vi "Update Generation On The Fly Digital Audio Task.vi"(7 "output level units":T1, 8 "error in (no error)":errorcluster, 10 "sine wave properties":T2, 11 "data task":T3) -> (0 "error out":errorcluster, 3 "data task":T3)   [LabVIEW 2021, in "DigitalAudioGenerationProcess.lvlib"]
uses:
  DigitalAudioGenerationProcess.lvlib
  <vilib>/PDM Acquisition Toolkit/host/Classes/Tasks/PCM Output/Controls/PCM Output Task DVR.ctl
  <vilib>/PDM Acquisition Toolkit/host/Classes/Tasks/PCM Output/PCM Output Task.lvclass
  C:/Program Files/National Instruments/LabVIEW 2021/vi.lib/PDM Acquisition Toolkit/host/Classes/Tasks/Parent/DecoderTask.lvclass
  controls/sine wave properties.ctl
  <vilib>/PDM Acquisition Toolkit/host/Classes/Channels/PCM Output/PCM Output Channel.lvclass
  C:/Program Files/National Instruments/LabVIEW 2021/vi.lib/PDM Acquisition Toolkit/host/Classes/Channels/DecoderChannel.lvclass
  <vilib>/PDM Acquisition Toolkit/host/Classes/Channels/PCM Output/controls/PCM Output Channel - Signal Properties.ctl
  <vilib>/PDM Acquisition Toolkit/host/Classes/Channels/DecoderChannel.lvclass
  C:/Program Files/National Instruments/LabVIEW 2021/vi.lib/PDM Acquisition Toolkit/host/Classes/Channels/PCM Output/PCM Output Channel.lvclass
  controls/AudioGenTypeDefs.lvlib
  shared/controls/digital output level units.ctl
  shared/controls/audio controls.lvlib
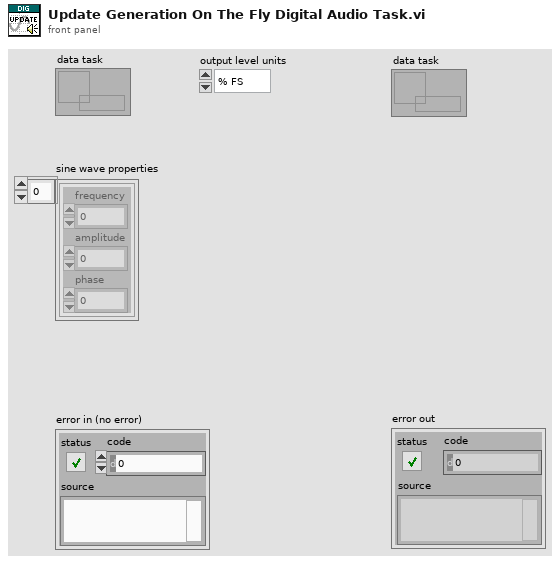
[diagram p1: front panel]
types:
  T1 = typedef "audio controls.lvlib/digital output level units.ctl" = enum32{"% FS", "dBFS", "V"}
  T2 = typedef "AudioGenTypeDefs.lvlib/sine wave properties.ctl" = cluster{"frequency":dbl, "amplitude":dbl, "phase":dbl}[]
  T3 = typedef "PDM Acquisition Class Library.lvlib/PCM Output Task.lvclass/PCM Output Task DVR.ctl" = refnum<data-value>
  T4 = typedef "PDM Acquisition Class Library.lvlib/PCM Output Channel.lvclass/PCM Output Channel - Signal Properties.ctl" = cluster{"cyclic period":dbl, "cyclic phase offset":dbl, "gain":dbl}
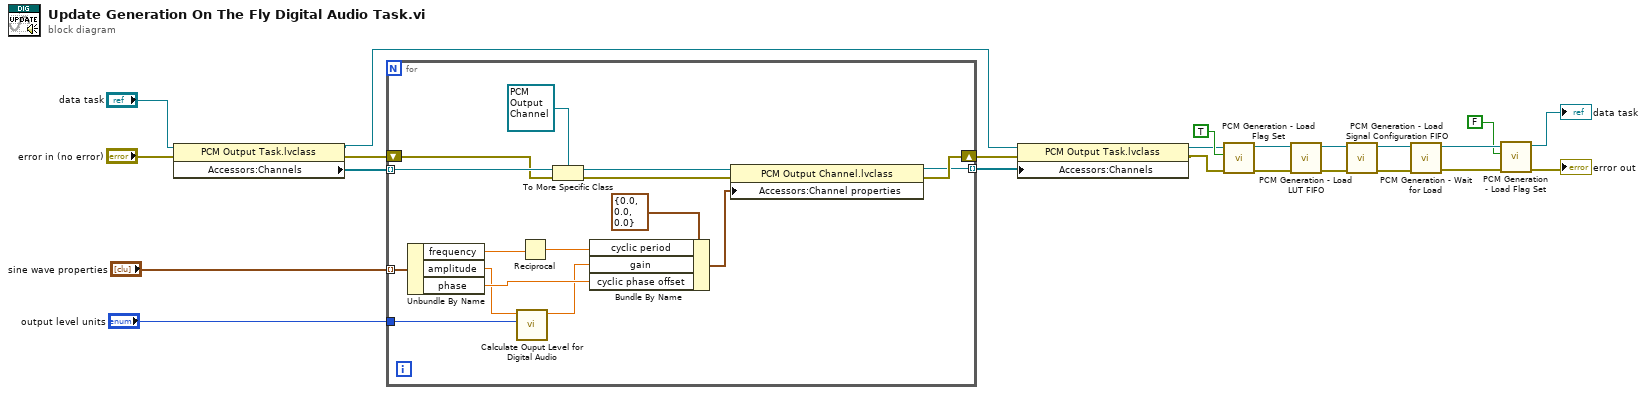
[diagram p0: block diagram]
diagram:
  n1 = property class="PCM Output Task.lvclass"(reference="data task", error in="error in (no error)") -> (reference out=w10:T3, error out=w22:errorcluster, "Accessors:Channels"=w23:refnum<class "DecoderChannel.lvclass">[])
  n2 = for {
    tunnel: w23 -> [w38] mode=indexing
    shift-right: [w34] -> w12
    shift-left: w22 -> [w36]
    tunnel: [w33] -> w11 mode=indexing
    tunnel: "sine wave properties" -> [w29] mode=indexing
    tunnel: "output level units" -> [w24]
    n3 = Unbundle By Name(w29) -> ("frequency"=w28:dbl, "amplitude"=w26:dbl, "phase"=w27:dbl)
    n4 = call "Calculate Ouput Level for Digital Audio.vi"("digital output level units"=w24, "output level"=w26) -> ("gain"=w25:dbl)  [unwired: 8 in, 1 out]
    n5 = Reciprocal(x=w28) -> (1/x=w32:dbl)
    n6 = To More Specific Class(target class=refnum<class "PCM Output Channel.lvclass"> refnum ("PDM Acquisition Class Library.lvlib:PCM Output Channel.lvclass"), reference=w38, error in=w36) -> (specific class reference=w35:refnum<class "PCM Output Channel.lvclass">, error out=w39:errorcluster)
    n7 = Bundle By Name(cluster=T4 {"cyclic period"=0.0, "cyclic phase offset"=0.0, "gain"=0.0} ("Channel properties"), "cyclic period"=w32, "gain"=w25, "cyclic phase offset"=w27) -> (w30:T4)
    n8 = property class="PCM Output Channel.lvclass"(reference=w35, error in=w39, "Accessors:Channel properties"=w30) -> (reference out=w33:refnum<class "PCM Output Channel.lvclass">, error out=w34:errorcluster)
  }
  n9 = property class="PCM Output Task.lvclass"(reference=w10, error in=w12, "Accessors:Channels"=w11) -> (reference out=w9:T3, error out=w8:errorcluster)
  n10 = call <vilib>:"PCM Generation - Load Flag Set.vi"("error in"=w8, "Load"=TRUE, "PCM Output Task In"=w9) -> ("error out"=w16:errorcluster, "PCM Output Task Out"=w15:T3)  [unwired: 7 in]
  n11 = call <vilib>:"PCM Generation - Load LUT FIFO.vi"("error in"=w16, "PCM Output Task In"=w15) -> ("error out"=w13:errorcluster, "PCM Output Task Out"=w14:T3)  [unwired: 8 in]
  n12 = call <vilib>:"PCM Generation - Load Signal Configuration FIFO.vi"("error in"=w13, "PCM Output Task In"=w14) -> ("error out"=w7:errorcluster, "PCM Output Task Out"=w17:T3)  [unwired: 8 in]
  n13 = call <vilib>:"PCM Generation - Wait for Load.vi"("error in"=w7, "PCM Output Task In"=w17) -> ("error out"=w19:errorcluster, "PCM Output Task Out"=w20:T3)  [unwired: 7 in, 1 out]
  n14 = call <vilib>:"PCM Generation - Load Flag Set.vi"("error in"=w19, "Load"=FALSE, "PCM Output Task In"=w20) -> ("error out"=→"error out":errorcluster, "PCM Output Task Out"=→"data task":T3)  [unwired: 7 in]
